vi "Translator DHTxx.vi"(0 "Input":variant, 11 "error in (no error)":errorcluster) -> (4 "Output":variant, 15 "error out":errorcluster)   [LabVIEW 2014, in "ESP8266 WiFi Wrapper.lvlib"]
doc: "An example of how to create the Translator to convert the LabVIEW VIs to Arduino C code."
uses:
  ESP8266 WiFi Wrapper.lvlib
panel:
  out "Outputs":string[](array[string])
  out "Inputs":string[](array[string])
  out "Output Datatypes":string[](array[string])
  out "Input Datatypes":string[](array[string])
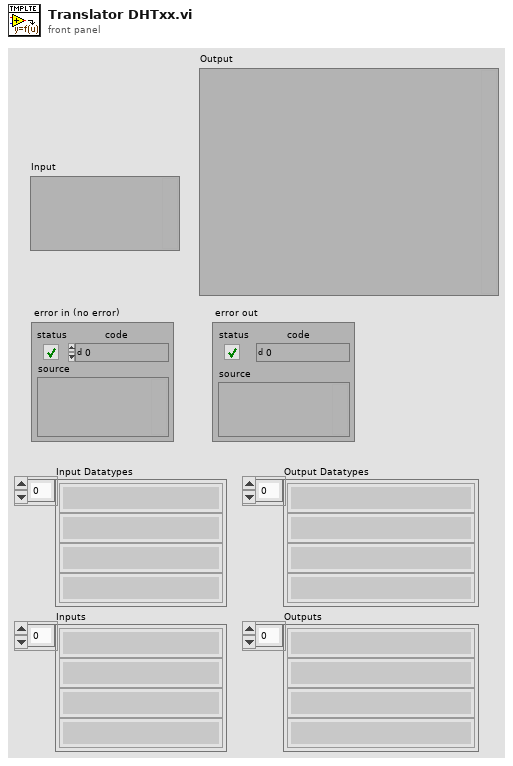
[diagram p1: front panel]
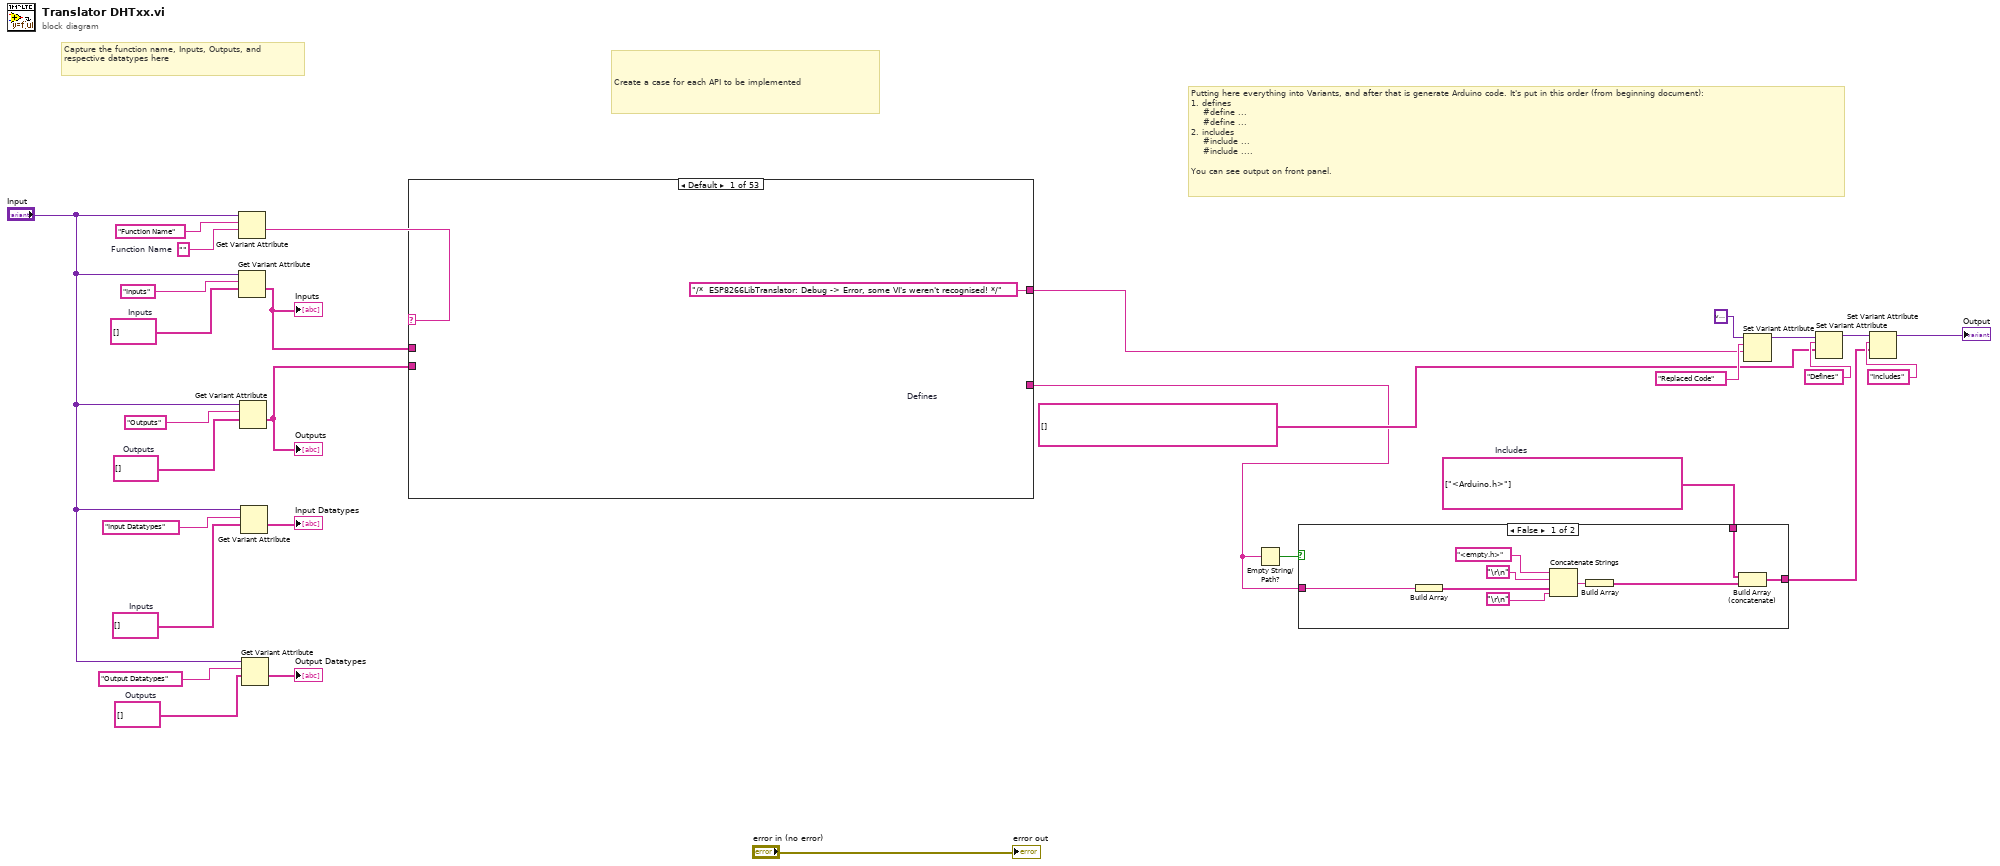
[diagram p0: block diagram]
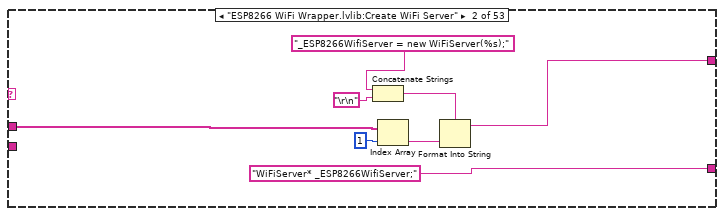
[diagram p3: hidden frame]
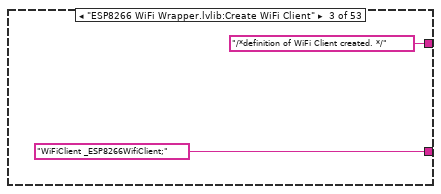
[diagram p4: hidden frame]
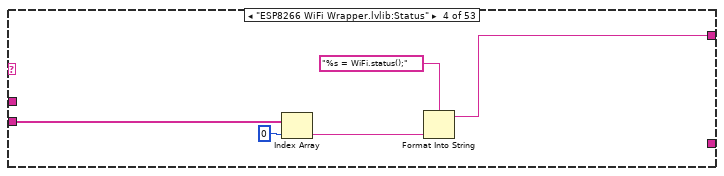
[diagram p5: hidden frame]
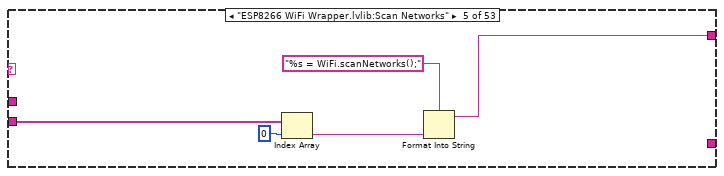
[diagram p6: hidden frame]
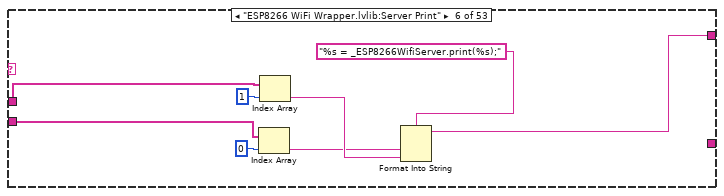
[diagram p7: hidden frame]
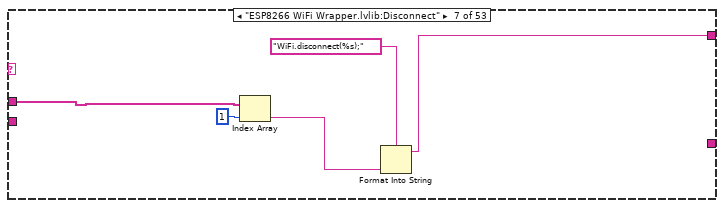
[diagram p8: hidden frame]
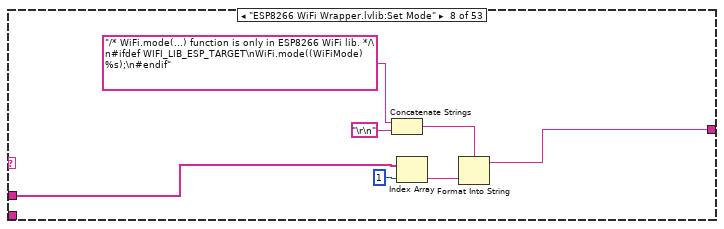
[diagram p9: hidden frame]
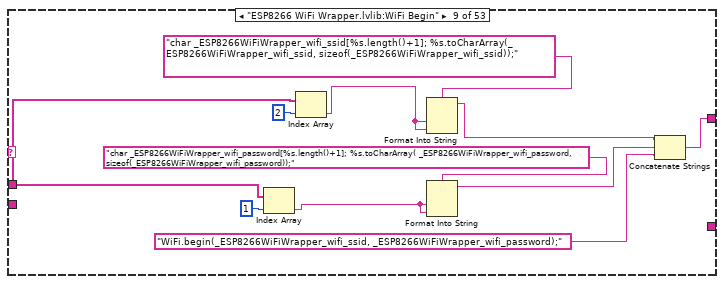
[diagram p10: hidden frame]
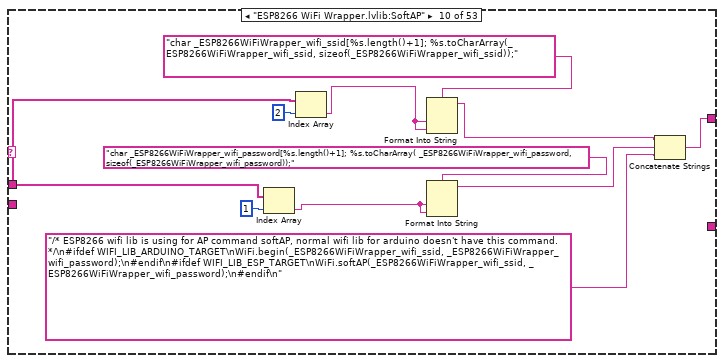
[diagram p11: hidden frame]
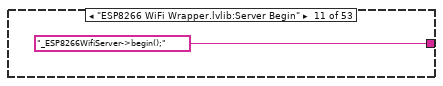
[diagram p12: hidden frame]
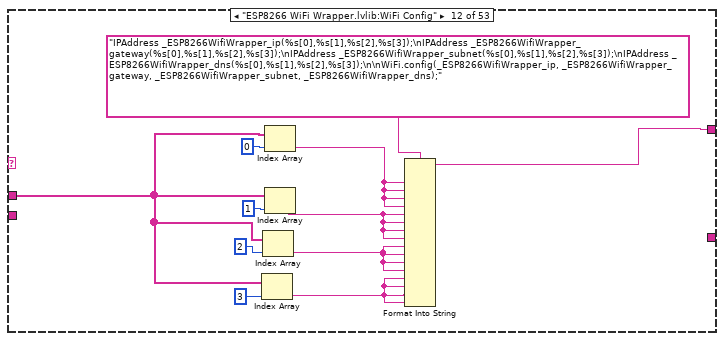
[diagram p13: hidden frame]
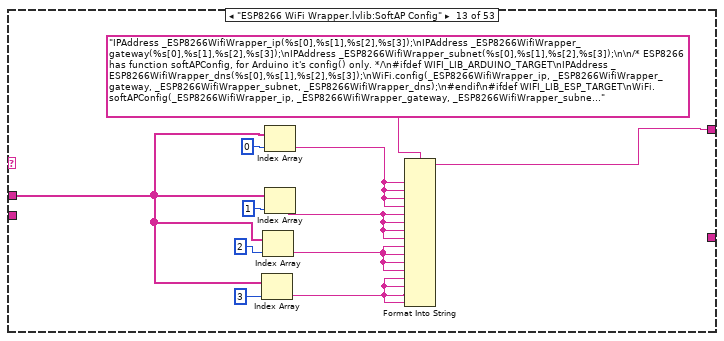
[diagram p14: hidden frame]
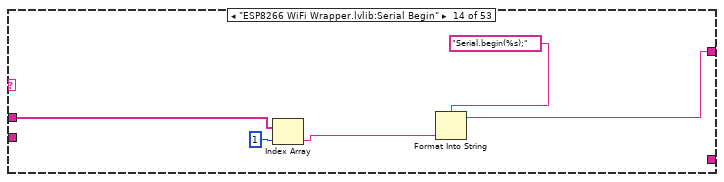
[diagram p15: hidden frame]
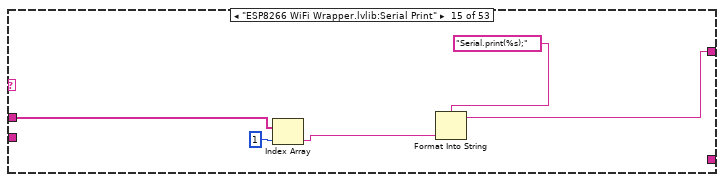
[diagram p16: hidden frame]
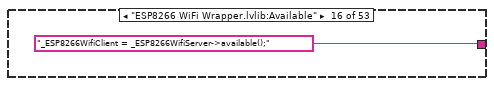
[diagram p17: hidden frame]
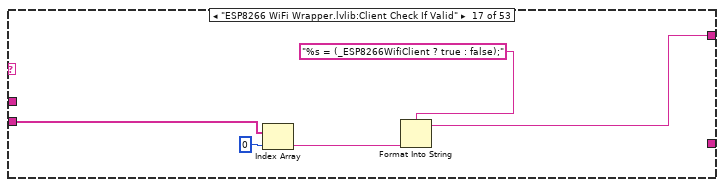
[diagram p18: hidden frame]
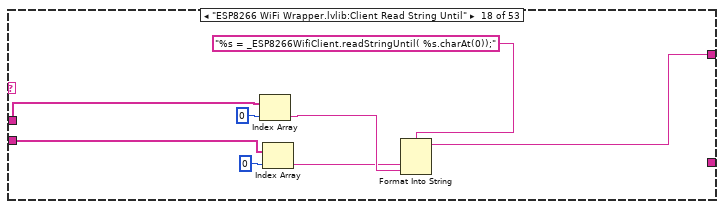
[diagram p19: hidden frame]
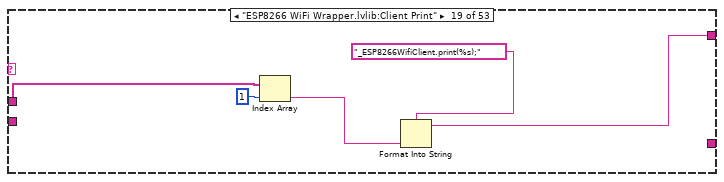
[diagram p20: hidden frame]
diagram:
  w4 = string[] []  # Defines
  w19 = string[] []  # Outputs
  w20 = string[] []  # Inputs
  w1 = string[] ["<Arduino.h>"]  # Includes
  w26 = string[] []  # Outputs
  w27 = string[] []  # Inputs
  w28 = ""  # Function Name
  # "Capture the function name, Inputs, Outputs, and respective datatypes here"
  # "Putting here everything into Variants, and after that is generate Arduino code. It's put in this order (from beginning document):\n1. defines\n    #define ...\n    #define ...\n2. includes\n    #include ...\n    #include ....\n\nYou can see output on front panel."
  # "Create a case for each API to be implemented"
  n1 = Get Variant Attribute(Variant="Input", name="Function Name", default value (empty Variant)=w28) -> (value=w10:string)  [unwired: 1 in, 3 out]
  n2 = Get Variant Attribute(Variant="Input", name="Inputs", default value (empty Variant)=w27) -> (value=w9:string[])  [unwired: 1 in, 3 out]
  "Inputs" <- w9
  n3 = Get Variant Attribute(Variant="Input", name="Outputs", default value (empty Variant)=w26) -> (value=w8:string[])  [unwired: 1 in, 3 out]
  "Outputs" <- w8
  n4 = Get Variant Attribute(Variant="Input", name="Input Datatypes", default value (empty Variant)=w20) -> (value=→"Input Datatypes":string[])  [unwired: 1 in, 3 out]
  n5 = Get Variant Attribute(Variant="Input", name="Output Datatypes", default value (empty Variant)=w19) -> (value=→"Output Datatypes":string[])  [unwired: 1 in, 3 out]
  n6 = case shown="Default" w10 {
    tunnel: w9 -> [_ w35 _ _ _ w56 w63 w66 w80 w91 _ w96 w107 w119 w124 _ _ w135 w142 w147 w152 w159 w170 _ _ w188 _ _ _ w206 w212 _ _ _ _ _ w252 w262 w269 _ _ w287 w297 _ _ _ _ _ _ w332 _ _ _]
    tunnel: w8 -> [_ _ _ w43 w48 w54 _ _ _ _ _ _ _ _ _ _ w131 w139 _ _ _ w156 w169 w177 w182 w191 _ w196 _ w205 w218 _ _ _ _ _ w250 w261 w273 w277 w280 w289 w296 w302 w307 w312 _ w318 w323 _ _ w343 w348]
    tunnel: ["/*  ESP8266LibTranslator: Debug -> Error, some VI's weren't recognised! */" w33 "/*definition of WiFi Client created. */" w42 w47 w58 w60 w65 w74 w85 "_ESP8266WifiServer->begin();" w101 w112 w117 w122 "_ESP8266WifiClient = _ESP8266WifiServer->available();" w128 w137 w144 w146 w151 w161 w172 w178 w181 w190 "_ESP8266WifiClient.stop();" w195 "_ESP8266WifiClient.flush();" w201 w214 "#ifdef WIFI_LIB_ESP_TARGET\nSerial.println( WiFi.softAPIP());\n#endif\n\n#ifdef WIFI_LIB_ARDUINO_TARGET\nSerial.println( WiFi.localIP());\n#endif" "Serial.println( WiFi.localIP());" w233 w241 "/*Debug -> WiFiUDP instance '_ESP8266WifiUDP' created.*/" w247 w264 w274 w275 w281 w290 w295 w301 w306 w311 "_ESP8266WifiUDP.flush();" w317 w322 w330 "ArduinoLabVIEW_DHT_1->begin();" w341 w346] -> w7
    tunnel: [_ "WiFiServer* _ESP8266WifiServer;" ("name") "WiFiClient _ESP8266WifiClient;" ("name") _ _ _ _ _ _ _ _ _ _ _ _ _ _ _ _ _ _ _ _ _ _ _ _ _ _ _ _ _ _ w229 w238 w242 _ _ _ _ _ _ _ _ _ _ _ _ _ "#include \"DHT.h\"\nDHT* ArduinoLabVIEW_DHT_1;" _ _ _] -> w3
    frame Default {
    }
    frame "ESP8266 WiFi Wrapper.lvlib:Create WiFi Server" {
      n7 = Concatenate Strings("_ESP8266WifiServer = new WiFiServer(%s);", "\r\n") -> (w38:string)
      n8 = Index Array(array=w35, index=1) -> (element=w36:string)
      n9 = Format Into String(format string=w38, w36) -> (resulting string=w33:string)  [unwired: 2 in, 1 out]
    }
    frame "ESP8266 WiFi Wrapper.lvlib:Create WiFi Client" {
    }
    frame "ESP8266 WiFi Wrapper.lvlib:Status" {
      n10 = Index Array(array=w43, index=0) -> (element=w45:string)
      n11 = Format Into String(format string="%s = WiFi.status();", w45) -> (resulting string=w42:string)  [unwired: 2 in, 1 out]
    }
    frame "ESP8266 WiFi Wrapper.lvlib:Scan Networks" {
      n12 = Index Array(array=w48, index=0) -> (element=w50:string)
      n13 = Format Into String(format string="%s = WiFi.scanNetworks();", w50) -> (resulting string=w47:string)  [unwired: 2 in, 1 out]
    }
    frame "ESP8266 WiFi Wrapper.lvlib:Server Print" {
      n14 = Index Array(array=w54, index=0) -> (element=w52:string)
      n15 = Index Array(array=w56, index=1) -> (element=w53:string)
      n16 = Format Into String(format string="%s = _ESP8266WifiServer.print(%s);", w52, w53) -> (resulting string=w58:string)  [unwired: 2 in, 1 out]
    }
    frame "ESP8266 WiFi Wrapper.lvlib:Disconnect" {
      n17 = Index Array(array=w63, index=1) -> (element=w62:string)
      n18 = Format Into String(format string="WiFi.disconnect(%s);", w62) -> (resulting string=w60:string)  [unwired: 2 in, 1 out]
    }
    frame "ESP8266 WiFi Wrapper.lvlib:Set Mode" {
      n19 = Concatenate Strings("/* WiFi.mode(...) function is only in ESP8266 WiFi lib. */\n#ifdef WIFI_LIB_ESP_TARGET\nWiFi.mode((WiFiMode) %s);\n#endif" ("name"), "\r\n") -> (w70:string)
      n20 = Index Array(array=w66, index=1) -> (element=w67:string)
      n21 = Format Into String(format string=w70, w67) -> (resulting string=w65:string)  [unwired: 2 in, 1 out]
    }
    frame "ESP8266 WiFi Wrapper.lvlib:WiFi Begin" {
      n22 = Index Array(array=w80, index=1) -> (element=w72:string)
      n23 = Index Array(array=w80, index=2) -> (element=w73:string)
      n24 = Format Into String(format string="char _ESP8266WiFiWrapper_wifi_ssid[%s.length()+1]; %s.toCharArray(_ESP8266WiFiWrapper_wifi_ssid, sizeof(_ESP8266WiFiWrapper_wifi_ssid));" ("name"), w73, w73) -> (resulting string=w77:string)  [unwired: 2 in, 1 out]
      n25 = Format Into String(format string="char _ESP8266WiFiWrapper_wifi_password[%s.length()+1]; %s.toCharArray( _ESP8266WiFiWrapper_wifi_password, sizeof(_ESP8266WiFiWrapper_wifi_password));" ("name"), w72, w72) -> (resulting string=w76:string)  [unwired: 2 in, 1 out]
      n26 = Concatenate Strings(w77, w76, "WiFi.begin(_ESP8266WiFiWrapper_wifi_ssid, _ESP8266WiFiWrapper_wifi_password);" ("name")) -> (w74:string)
    }
    frame "ESP8266 WiFi Wrapper.lvlib:SoftAP" {
      n27 = Index Array(array=w91, index=1) -> (element=w83:string)
      n28 = Index Array(array=w91, index=2) -> (element=w84:string)
      n29 = Format Into String(format string="char _ESP8266WiFiWrapper_wifi_ssid[%s.length()+1]; %s.toCharArray(_ESP8266WiFiWrapper_wifi_ssid, sizeof(_ESP8266WiFiWrapper_wifi_ssid));" ("name"), w84, w84) -> (resulting string=w88:string)  [unwired: 2 in, 1 out]
      n30 = Format Into String(format string="char _ESP8266WiFiWrapper_wifi_password[%s.length()+1]; %s.toCharArray( _ESP8266WiFiWrapper_wifi_password, sizeof(_ESP8266WiFiWrapper_wifi_password));" ("name"), w83, w83) -> (resulting string=w87:string)  [unwired: 2 in, 1 out]
      n31 = Concatenate Strings(w88, w87, "/* ESP8266 wifi lib is using for AP command softAP, normal wifi lib for arduino doesn't have this command. */\n#ifdef WIFI_LIB_ARDUINO_TARGET\nWiFi.begin(_ESP8266WiFiWrapper_wifi_ssid, _ESP8266WiFiWrapper_wifi_password);\n#endif\n#ifdef WIFI_LIB_ESP_TARGET\nWiFi.softAP(_ESP8266WiFiWrapper_wifi_ssid, _ESP8266WiFiWrapper_wifi_password);\n#endif\n" ("name")) -> (w85:string)
    }
    frame "ESP8266 WiFi Wrapper.lvlib:Server Begin" {
    }
    frame "ESP8266 WiFi Wrapper.lvlib:WiFi Config" {
      n32 = Index Array(array=w96, index=3) -> (element=w95:string)
      n33 = Index Array(array=w96, index=2) -> (element=w100:string)
      n34 = Index Array(array=w96, index=0) -> (element=w98:string)
      n35 = Index Array(array=w96, index=1) -> (element=w99:string)
      n36 = Format Into String(format string="IPAddress _ESP8266WifiWrapper_ip(%s[0],%s[1],%s[2],%s[3]);\nIPAddress _ESP8266WifiWrapper_gateway(%s[0],%s[1],%s[2],%s[3]);\nIPAddress _ESP8266WifiWrapper_subnet(%s[0],%s[1],%s[2],%s[3]);\nIPAddress _ESP8266WifiWrapper_dns(%s[0],%s[1],%s[2],%s[3]);\n\nWiFi.config(_ESP8266WifiWrapper_ip, _ESP8266WifiWrapper_gateway, _ESP8266WifiWrapper_subnet, _ESP8266WifiWrapper_dns);", w98, w98, w98, w98, w99, w99, w99, w99, w100, w100, w100, w100, w95, w95, w95, w95) -> (resulting string=w101:string)  [unwired: 2 in, 1 out]
    }
    frame "ESP8266 WiFi Wrapper.lvlib:SoftAP Config" {
      n37 = Index Array(array=w107, index=3) -> (element=w106:string)
      n38 = Index Array(array=w107, index=2) -> (element=w111:string)
      n39 = Index Array(array=w107, index=0) -> (element=w109:string)
      n40 = Index Array(array=w107, index=1) -> (element=w110:string)
      n41 = Format Into String(format string="IPAddress _ESP8266WifiWrapper_ip(%s[0],%s[1],%s[2],%s[3]);\nIPAddress _ESP8266WifiWrapper_gateway(%s[0],%s[1],%s[2],%s[3]);\nIPAddress _ESP8266WifiWrapper_subnet(%s[0],%s[1],%s[2],%s[3]);\n\n/* ESP8266 has function softAPConfig, for Arduino it's config() only. */\n#ifdef WIFI_LIB_ARDUINO_TARGET\nIPAddress _ESP8266WifiWrapper_dns(%s[0],%s[1],%s[2],%s[3]);\nWiFi.config(_ESP8266WifiWrapper_ip, _ESP8266WifiWrapper_gateway, _ESP8266WifiWrapper_subnet, _ESP8266WifiWrapper_dns);\n#endif\n#ifdef WIFI_LIB_ESP_TARGET\nWiFi.softAPConfig(_ESP8266WifiWrapper_ip, _ESP8266WifiWrapper_gateway, _ESP8266WifiWrapper_subnet);\n#endif", w109, w109, w109, w109, w110, w110, w110, w110, w111, w111, w111, w111, w106, w106, w106, w106) -> (resulting string=w112:string)  [unwired: 2 in, 1 out]
    }
    frame "ESP8266 WiFi Wrapper.lvlib:Serial Begin" {
      n42 = Index Array(array=w119, index=1) -> (element=w120:string)
      n43 = Format Into String(format string="Serial.begin(%s);", w120) -> (resulting string=w117:string)  [unwired: 2 in, 1 out]
    }
    frame "ESP8266 WiFi Wrapper.lvlib:Serial Print" {
      n44 = Index Array(array=w124, index=1) -> (element=w125:string)
      n45 = Format Into String(format string="Serial.print(%s);", w125) -> (resulting string=w122:string)  [unwired: 2 in, 1 out]
    }
    frame "ESP8266 WiFi Wrapper.lvlib:Available" {
    }
    frame "ESP8266 WiFi Wrapper.lvlib:Client Check If Valid" {
      n46 = Index Array(array=w131, index=0) -> (element=w129:string)
      n47 = Format Into String(format string="%s = (_ESP8266WifiClient ? true : false);", w129) -> (resulting string=w128:string)  [unwired: 2 in, 1 out]
    }
    frame "ESP8266 WiFi Wrapper.lvlib:Client Read String Until" {
      n48 = Index Array(array=w135, index=0) -> (element=w134:string)
      n49 = Index Array(array=w139, index=0) -> (element=w133:string)
      n50 = Format Into String(format string="%s = _ESP8266WifiClient.readStringUntil( %s.charAt(0));", w133, w134) -> (resulting string=w137:string)  [unwired: 2 in, 1 out]
    }
    frame "ESP8266 WiFi Wrapper.lvlib:Client Print" {
      n51 = Index Array(array=w142, index=1) -> (element=w141:string)
      n52 = Format Into String(format string="_ESP8266WifiClient.print(%s);", w141) -> (resulting string=w144:string)  [unwired: 2 in, 1 out]
    }
    frame "ESP8266 WiFi Wrapper.lvlib:Client Println" {
      n53 = Index Array(array=w147, index=1) -> (element=w150:string)
      n54 = Format Into String(format string="_ESP8266WifiClient.println(%s);", w150) -> (resulting string=w146:string)  [unwired: 2 in, 1 out]
    }
    frame "ESP8266 WiFi Wrapper.lvlib:Client Write" {
      n55 = Index Array(array=w152, index=1) -> (element=w153:string)
      n56 = Format Into String(format string="_ESP8266WifiClient.write(%s);", w153) -> (resulting string=w151:string)  [unwired: 2 in, 1 out]
    }
    frame "ESP8266 WiFi Wrapper.lvlib:Client Connect To IP" {
      n57 = Index Array(array=w159, index=1) -> (element=w158:string)
      n58 = Index Array(array=w159, index=0) -> (element=w162:string)
      n59 = Index Array(array=w156, index=0) -> (element=w157:string)
      n60 = Format Into String(format string="%s = _ESP8266WifiClient.connect(IPAddress(%s[0],%s[1],%s[2],%s[3]), %s);", w157, w158, w158, w158, w158, w162) -> (resulting string=w161:string)  [unwired: 2 in, 1 out]
    }
    frame "ESP8266 WiFi Wrapper.lvlib:Client Connect To URL" {
      n61 = Index Array(array=w169, index=0) -> (element=w168:string)
      n62 = Index Array(array=w170, index=1) -> (element=w167:string)
      n63 = Index Array(array=w170, index=0) -> (element=w166:string)
      n64 = Format Into String(format string="char _ESP8266WiFiWrapper_clientUrl[%s.length()+1]; %s.toCharArray(_ESP8266WiFiWrapper_clientUrl, sizeof(_ESP8266WiFiWrapper_clientUrl));\n%s = _ESP8266WifiClient.connect(_ESP8266WiFiWrapper_clientUrl, %s);", w167, w167, w168, w166) -> (resulting string=w172:string)  [unwired: 2 in, 1 out]
    }
    frame "ESP8266 WiFi Wrapper.lvlib:Client Is Connected" {
      n65 = Index Array(array=w177, index=0) -> (element=w176:string)
      n66 = Format Into String(format string="%s = _ESP8266WifiClient.connected();", w176) -> (resulting string=w178:string)  [unwired: 2 in, 1 out]
    }
    frame "ESP8266 WiFi Wrapper.lvlib:Client Read" {
      n67 = Index Array(array=w182, index=0) -> (element=w183:string)
      n68 = Format Into String(format string="%s = _ESP8266WifiClient.read();", w183) -> (resulting string=w181:string)  [unwired: 2 in, 1 out]
    }
    frame "ESP8266 WiFi Wrapper.lvlib:Client Read Bytes" {
      n69 = Index Array(array=w191, index=0) -> (element=w187:string)
      n70 = Index Array(array=w188, index=1) -> (element=w186:string)
      n71 = Format Into String(format string="%s = _ESP8266WifiClient.read(%s.ptr(), %s.size());", w187, w186, w186) -> (resulting string=w190:string)  [unwired: 2 in, 1 out]
    }
    frame "ESP8266 WiFi Wrapper.lvlib:Client Stop" {
    }
    frame "ESP8266 WiFi Wrapper.lvlib:Client Available" {
      n72 = Index Array(array=w196, index=0) -> (element=w199:string)
      n73 = Format Into String(format string="%s = _ESP8266WifiClient.available();", w199) -> (resulting string=w195:string)  [unwired: 2 in, 1 out]
    }
    frame "ESP8266 WiFi Wrapper.lvlib:Client Flush" {
      # "Here would be also handling which instance has to read, there is INPUT parameter\ninstance ID. These function are in development. There would be factory producer\nfor Client instances."
    }
    frame "ESP8266 WiFi Wrapper.lvlib:String Index Of" {
      n74 = Index Array(array=w206, index=2) -> (element=w203:string)
      n75 = Index Array(array=w206, index=0) -> (element=w202:string)
      n76 = Index Array(array=w205, index=0) -> (element=w204:string)
      n77 = Format Into String(format string="%s = %s.indexOf(%s);", w204, w203, w202) -> (resulting string=w201:string)  [unwired: 2 in, 1 out]
    }
    frame "ESP8266 WiFi Wrapper.lvlib:String Index Of From" {
      n78 = Index Array(array=w212, index=3) -> (element=w216:string)
      n79 = Index Array(array=w212, index=0) -> (element=w211:string)
      n80 = Index Array(array=w212, index=1) -> (element=w215:string)
      n81 = Index Array(array=w218, index=0) -> (element=w217:string)
      n82 = Format Into String(format string="%s = %s.indexOf(%s, %s);", w217, w216, w215, w211) -> (resulting string=w214:string)  [unwired: 2 in, 1 out]
    }
    frame "ESP8266 WiFi Wrapper.lvlib:Serial Wifi Print SoftAPIP" {
    }
    frame "ESP8266 WiFi Wrapper.lvlib:Serial Wifi Print IP" {
      (unwired) "#ifdef WIFI_LIB_ESP_TARGET\nSerial.println( WiFi.softAPIP());\n#endif\n\n#ifdef WIFI_LIB_ARDUINO_TARGET\nSerial.println( WiFi.localIP());\n#endif"
    }
    frame "ESP8266 WiFi Wrapper.lvlib:Arduino Target" {
      w226 = "\r\n"
      # "SPI is needed for Arduino WiFi lib. It's included in other header\nfiles, but cores libs have to be included in main sketch!!!\nFamous IDE feature. Read on internet about that, I spent few\nhours until figured out about that :D"
      # "If target is set up for Arduino, it has to include library for it."
      n83 = Concatenate Strings("/*including header file for Arduino target */" ("string"), w226, "#define WIFI_LIB_ARDUINO_TARGET" ("string"), w226, "#include <SPI.h>" ("name"), w226, "#include <WiFi.h>" ("name")) -> (w229:string)
      n84 = Concatenate Strings("/*  Debug -> Target device changed to Arduino, including WiFi.h file, look at beginning of file. */" ("string"), "\r\n") -> (w233:string)
    }
    frame "ESP8266 WiFi Wrapper.lvlib:ESP Target" {
      w235 = "\r\n"
      # "If target is set up for ESP, it has to include library for it."
      n85 = Concatenate Strings("/*including header file for ESP target */" ("string"), w235, "#define WIFI_LIB_ESP_TARGET" ("string"), w235, "#include <ESP8266WiFi.h>" ("name")) -> (w238:string)
      n86 = Concatenate Strings("/* Debug -> Target device changed to ESP, including ESP8266WiFi.h file, look at beginning of file. */" ("string"), "\r\n") -> (w241:string)
    }
    frame "ESP8266 WiFi Wrapper.lvlib:Create UDP" {
      n87 = Concatenate Strings("#include <WiFiUdp.h>" ("name"), "\r\n", "WiFiUDP _ESP8266WifiUDP;" ("name")) -> (w242:string)
    }
    frame "ESP8266 WiFi Wrapper.lvlib:UDP Begin" {
      n88 = Index Array(array=w252, index=1) -> (element=w249:string)
      n89 = Index Array(array=w250, index=0) -> (element=w248:string)
      n90 = Format Into String(format string="%s = _ESP8266WifiUDP.begin(%s);", w248, w249) -> (resulting string=w247:string)  [unwired: 2 in, 1 out]
    }
    frame "ESP8266 WiFi Wrapper.lvlib:UDP Begin Packet URL" {
      n91 = Index Array(array=w262, index=0) -> (element=w255:string)
      n92 = Index Array(array=w261, index=0) -> (element=w256:string)
      n93 = Index Array(array=w262, index=2) -> (element=w257:string)
      n94 = Format Into String(format string="char _ESP8266WiFiWrapper_packetRemoteURL[%s.length()+1]; %s.toCharArray(_ESP8266WiFiWrapper_packetRemoteURL, sizeof(_ESP8266WiFiWrapper_packetRemoteURL));\n%s = _ESP8266WifiUDP.beginPacket(_ESP8266WiFiWrapper_packetRemoteURL, %s);", w257, w257, w256, w255) -> (resulting string=w264:string)  [unwired: 2 in, 1 out]
    }
    frame "ESP8266 WiFi Wrapper.lvlib:UDP Begin Packet IP" {
      n95 = Index Array(array=w273, index=0) -> (element=w265:string)
      n96 = Index Array(array=w269, index=2) -> (element=w266:string)
      n97 = Index Array(array=w269, index=0) -> (element=w268:string)
      n98 = Format Into String(format string="%s = _ESP8266WifiUDP.beginPacket(IPAddress(%s[0],%s[1],%s[2],%s[3]), %s);", w265, w266, w266, w266, w266, w268) -> (resulting string=w274:string)  [unwired: 2 in, 1 out]
    }
    frame "ESP8266 WiFi Wrapper.lvlib:UDP Available" {
      n99 = Index Array(array=w277, index=0) -> (element=w276:string)
      n100 = Format Into String(format string="%s = _ESP8266WifiUDP.available();", w276) -> (resulting string=w275:string)  [unwired: 2 in, 1 out]
    }
    frame "ESP8266 WiFi Wrapper.lvlib:UDP End Packet" {
      n101 = Index Array(array=w280, index=0) -> (element=w282:string)
      n102 = Format Into String(format string="%s = _ESP8266WifiUDP.endPacket();", w282) -> (resulting string=w281:string)  [unwired: 2 in, 1 out]
    }
    frame "ESP8266 WiFi Wrapper.lvlib:UDP Write Byte" {
      n103 = Index Array(array=w287, index=1) -> (element=w285:string)
      n104 = Index Array(array=w289, index=0) -> (element=w286:string)
      n105 = Format Into String(format string="%s = _ESP8266WifiUDP.write(%s);", w286, w285) -> (resulting string=w290:string)  [unwired: 2 in, 1 out]
    }
    frame "ESP8266 WiFi Wrapper.lvlib:UDP Write String" {
      n106 = Index Array(array=w297, index=1) -> (element=w294:string)
      n107 = Index Array(array=w296, index=0) -> (element=w293:string)
      n108 = Format Into String(format string="char _ESP8266WiFiWrapper_UDPWriteString[%s.length()+1]; %s.toCharArray(_ESP8266WiFiWrapper_UDPWriteString, sizeof(_ESP8266WiFiWrapper_UDPWriteString));\n%s = _ESP8266WifiUDP.write( _ESP8266WiFiWrapper_UDPWriteString);", w294, w294, w293) -> (resulting string=w295:string)  [unwired: 2 in, 1 out]
    }
    frame "ESP8266 WiFi Wrapper.lvlib:UDP Parse Packet" {
      n109 = Index Array(array=w302, index=0) -> (element=w303:string)
      n110 = Format Into String(format string="%s = _ESP8266WifiUDP.parsePacket();", w303) -> (resulting string=w301:string)  [unwired: 2 in, 1 out]
    }
    frame "ESP8266 WiFi Wrapper.lvlib:UDP Peek" {
      n111 = Index Array(array=w307, index=0) -> (element=w308:string)
      n112 = Format Into String(format string="%s = _ESP8266WifiUDP.peek();", w308) -> (resulting string=w306:string)  [unwired: 2 in, 1 out]
    }
    frame "ESP8266 WiFi Wrapper.lvlib:UDP Read" {
      n113 = Index Array(array=w312, index=0) -> (element=w313:string)
      n114 = Format Into String(format string="%s = _ESP8266WifiUDP.read();", w313) -> (resulting string=w311:string)  [unwired: 2 in, 1 out]
    }
    frame "ESP8266 WiFi Wrapper.lvlib:UDP Flush" {
    }
    frame "ESP8266 WiFi Wrapper.lvlib:UDP Remote IP to String" {
      n115 = Index Array(array=w318, index=0) -> (element=w319:string)
      n116 = Format Into String(format string="%s = (String) _ESP8266WifiUDP.remoteIP();", w319) -> (resulting string=w317:string)  [unwired: 2 in, 1 out]
    }
    frame "ESP8266 WiFi Wrapper.lvlib:UDP Remote Port" {
      n117 = Index Array(array=w323, index=0) -> (element=w324:string)
      n118 = Format Into String(format string="%s = _ESP8266WifiUDP.remotePort();", w324) -> (resulting string=w322:string)  [unwired: 2 in, 1 out]
    }
    frame "ESP8266 WiFi Wrapper.lvlib:DHTxx Create" {
      n119 = Concatenate Strings("char DHTxx_auxTypeVar = %s;" ("name"), "\r\n", "if (DHTxx_auxTypeVar == 0) DHTxx_auxTypeVar = 11;\nif (DHTxx_auxTypeVar == 1) DHTxx_auxTypeVar = 21;\nif (DHTxx_auxTypeVar == 2) DHTxx_auxTypeVar = 22;" ("name"), "\r\n", "ArduinoLabVIEW_DHT_1 = new DHT( %s, DHTxx_auxTypeVar);" ("name")) -> (w337:string)
      n120 = Index Array(array=w332, index #1=0 ("index"), index #2=2 ("index")) -> (element #1=w333:string, element #2=w334:string)
      n121 = Format Into String(format string=w337, w333, w334) -> (resulting string=w330:string)  [unwired: 2 in, 1 out]
    }
    frame "ESP8266 WiFi Wrapper.lvlib:DHTxx Begin" {
    }
    frame "ESP8266 WiFi Wrapper.lvlib:DHTxx Read Temperature" {
      n122 = Index Array(array=w343, index=0) -> (element=w344:string)
      n123 = Format Into String(format string="%s = ArduinoLabVIEW_DHT_1->readTemperature();", w344) -> (resulting string=w341:string)  [unwired: 2 in, 1 out]
    }
    frame "ESP8266 WiFi Wrapper.lvlib:DHTxx Read Humidity" {
      n124 = Index Array(array=w348, index=0) -> (element=w349:string)
      n125 = Format Into String(format string="%s = ArduinoLabVIEW_DHT_1->readHumidity();", w349) -> (resulting string=w346:string)  [unwired: 2 in, 1 out]
    }
  }
  n126 = Empty String/Path?(string/path=w3) -> (empty?=w5:bool)
  n127 = case shown="False" w5 {
    tunnel: w3 -> [w359 _]
    tunnel: [w352 w360] -> w2
    tunnel: w1 -> [w351 w360]
    frame False {
      n128 = Build Array(w359) -> (w353:string[])
      n129 = Concatenate Strings("<empty.h>" ("string"), "\r\n", w353, "\r\n") -> (w354:string)
      n130 = Build Array(w354) -> (w358:string[])
      n131 = Build Array (concatenate)(w351, w358) -> (w352:string[])
    }
    frame True {
    }
  }
  n132 = Set Variant Attribute(Variant=variant ("variant"), name="Replaced Code", value=w7) -> (Variant out=w13:variant)  [unwired: 1 in, 2 out]
  n133 = Set Variant Attribute(Variant=w13, name="Defines", value=w4) -> (Variant out=w12:variant)  [unwired: 1 in, 2 out]
  n134 = Set Variant Attribute(Variant=w12, name="Includes", value=w2) -> (Variant out=→"Output":variant)  [unwired: 1 in, 2 out]
  "error out" <- "error in (no error)"
